vi "rwr_Connect to Server.vi"(4 "Show in Debugger?":bool=TRUE, 6 "Message Priority":T1=enum."Normal", 7 "Caller in":refnum<class "Worker.lvclass">, 8 "error in":errorcluster, 9 "timeout (ms)":i32=30000, 10 "Data in":T3, 11 "TCP Client in":refnum<class "TCP Client.lvclass">) -> (0 "error out":errorcluster, 2 "Reply Data out":T2, 3 "dup TCP Client out":refnum<class "TCP Client.lvclass">, 5 "dup Caller out":refnum<class "Worker.lvclass">)   [LabVIEW 2017, in "_TCP Client.lvlib" / "TCP Client.lvclass"]
doc: "This VI sends a <b>Public API Request with Reply</b> message to an MHL case of the Worker that owns this VI. This VI will wait until it receives a <b>Reply</b> message back from the Worker that owns this VI. If the wait time exceeds <b>timeout (ms)</b>, an error will be returned.\n---\nEstablish a connection a TCP Server. Return an error message if the connection could not be estabished."
uses:
  TCP Client.lvclass
  C:/SC/Source Code/VIPM/LabVIEW 20xx/vi.lib/addons/_Workers/Library/Classes/Worker/Worker.lvclass
  <vilib>/addons/_Workers/Library/Classes/Worker/Worker.lvclass
  rwr_Connect to Server.ctl
  rwr_Connect to Server Reply.ctl
  <vilib>/addons/_Workers/Library/Classes/Message/Priority.ctl
  <vilib>/addons/_Workers/Library/Case Label.ctl
  <vilib>/addons/_Workers/Library/Classes/Message Queue/Message Queue.lvclass
  <vilib>/addons/_Workers/Library/Workers.lvlib
  <vilib>/addons/_Workers/Library/Classes/Message/Message.lvclass
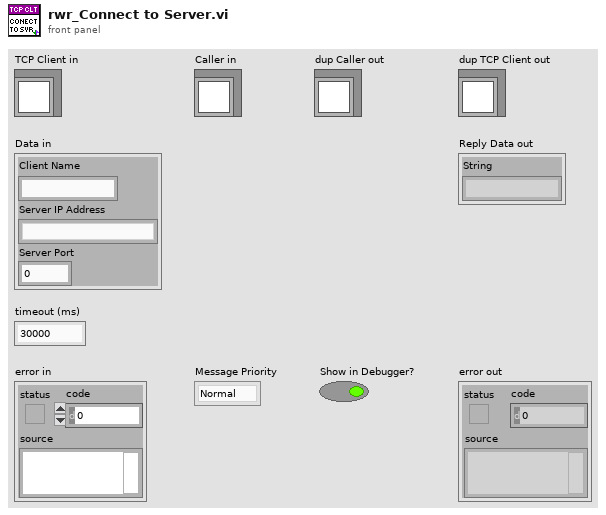
[diagram p1: front panel]
types:
  T1 = typedef "Workers.lvlib/Message.lvclass/Priority.ctl" = enum16{"Low", "Normal", "High"}
  T2 = typedef "_TCP Client.lvlib/TCP Client.lvclass/rwr_Connect to Server Reply.ctl" = cluster{"String":string}
  T3 = typedef "_TCP Client.lvlib/TCP Client.lvclass/rwr_Connect to Server.ctl" = cluster{"Client Name":string, "Server IP Address":string, "Server Port":u16}
  T4 = typedef "Workers.lvlib/Case Label.ctl" = string
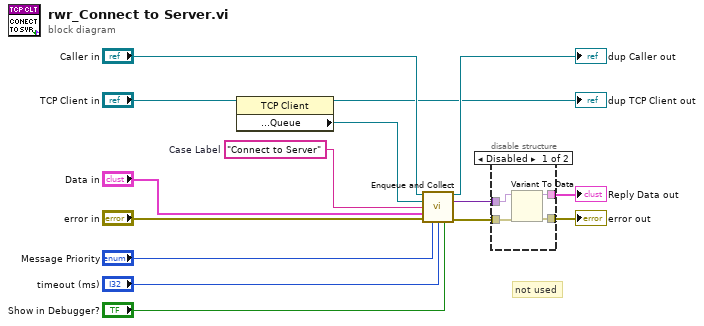
[diagram p0: block diagram]
diagram:
  w1 = T4 "Connect to Server"  # Case Label
  # "not used"
  n1 = property class="TCP Client"(reference="TCP Client in") -> (reference out=→"dup TCP Client out":refnum<class "TCP Client.lvclass">, "Accessors:Read:Public API:Queue"=w2:refnum<class "Message Queue.lvclass">)  [unwired: 1 in, 1 out]
  n2 = call-dynamic "Enqueue and Collect.vi"("Worker"="Caller in", "Message Queue"=w2, "Case Label"=w1, "Data"="Data in", "error in (no error)"="error in", "Priority (Normal)"="Message Priority", "timeout in ms"="timeout (ms)", "Send Message to Debugger? (T)"="Show in Debugger?") -> ("dup Worker out"=→"dup Caller out":refnum<class "Worker.lvclass">, "Data out"=w7:variant, "error out"=w8:errorcluster)  [unwired: 4 in, 1 out]
  n3 = disable-structure shown="Disabled" {
    disable-tunnel: [w19 w20] -> w14
    disable-tunnel: [w18 _] -> w13
    disable-tunnel: w8 -> [w17 w20]
    disable-tunnel: w7 -> [w16 _]
    frame Disabled {
      n4 = Variant To Data(error in=w17, Variant=w16) -> (data=w18:variant, error out=w19:errorcluster)  [unwired: 1 in]
    }
    frame Enabled {
    }
  }
  "error out" <- w14
  "Reply Data out" <- w13
